vi "Cursor Location.vi"(3 "Coordinates":cluster{"x (m)":dbl, "y (m)":dbl, "z (mm)":dbl} {"z (mm)" format="%.1f"; "y (m)" format="%.1p"; "x (m)" format="%.1p"}, 4 "Frame Properties (m)":T1) -> (0 "Y-Coordinate":dbl, 1 "X-Coordinate":dbl)   [LabVIEW 2022 SP3]
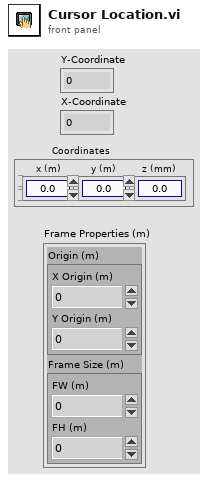
[diagram p1: front panel]
types:
  T1 = cluster{"Origin (m)":cluster{"X Origin (m)":dbl, "Y Origin (m)":dbl}, "Frame Size (m)":cluster{"FW (m)":dbl, "FH (m)":dbl}}
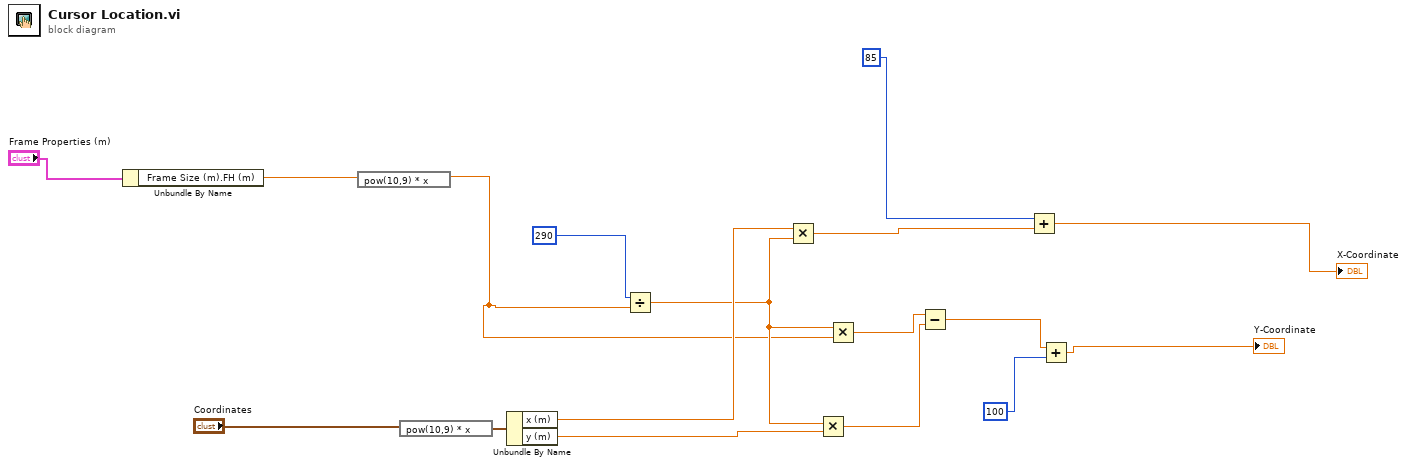
[diagram p0: block diagram]
diagram:
  n1 = Unbundle By Name("Frame Properties (m)") -> ("Frame Size (m).FH (m)"=w9:dbl)
  n2 = expression code="pow(10,9) * x"(w9) -> (w4:dbl)
  n3 = expression code="pow(10,9) * x"("Coordinates") -> (w17:cluster{"x (m)":dbl, "y (m)":dbl, "z (mm)":dbl})
  n4 = Unbundle By Name(w17) -> ("x (m)"=w15:dbl, "y (m)"=w14:dbl)
  n5 = Divide(x=290, y=w4) -> (x/y=w6:dbl)
  n6 = Multiply(x=w15, y=w6) -> (x*y=w13:dbl)
  n7 = Multiply(x=w6, y=w14) -> (x*y=w10:dbl)
  n8 = Multiply(x=w6, y=w4) -> (x*y=w5:dbl)
  n9 = Subtract(x=w5, y=w10) -> (x-y=w2:dbl)
  n10 = Add(x=85, y=w13) -> (x+y=→"X-Coordinate":dbl)
  n11 = Add(x=w2, y=100) -> (x+y=→"Y-Coordinate":dbl)
